vi "Get Connector Pane Info.vi"(8 "error in (no error)":errorcluster, 11 "vi reference":refnum<vi>) -> (0 "error out":errorcluster, 3 "Terminals":T1[](array[typedef]))   [LabVIEW 2020, in "MCP Server.lvlib"]
doc: "Utilizes the Application method \"Get ConPane Datatype\" to read the terminal properties of a subVI without loading it or requiring VI scripting."
uses:
  MCP Server.lvlib
  <vilib>/Utility/Data Type/NI_Data Type.lvlib
  Terminal.ctl
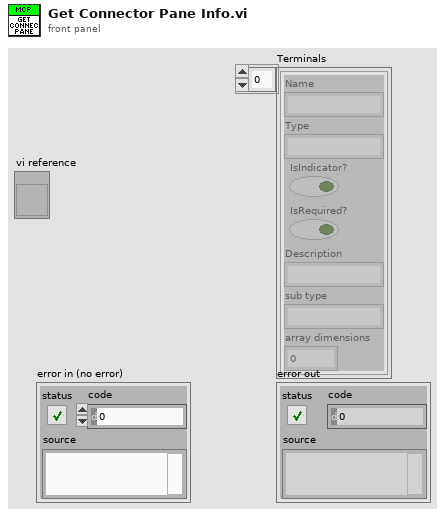
[diagram p1: front panel]
types:
  T1 = typedef "MCP Server.lvlib/Terminal.ctl" = cluster{"Name":string, "Type":string, "IsIndicator?":bool, "IsRequired?":bool, "Description":string, "sub type":string, "array dimensions":i32}
  T2 = typedef "NI_Data Type.lvlib/VI Info.ctl" = cluster{"Connector Pane Pattern":i16, "Connector Pane Rotation":i16, "Flags":u32[], "Modification Date":timestamp, "Asynchronous":bool, "Non-Function":bool, "Subroutine":bool, "SubSystem":bool}
  T3 = typedef "NI_Data Type.lvlib/Data Type.ctl" = enum8{"Invalid Type", "Void", "I8", "I16", "I32", "I64", "U8", "U16", "U32", "U64", "Single Float", "Double Float", "Extended Float", "Single Complex", "Double Complex", "Extended Complex", "Enum U8", "Enum U16", "Enum U32", "Enum U64", "Single Float With Unit", "Double Float With Unit", "Extended Float With Unit", "Single Complex with Unit", "Double Complex with Unit", "Extended Complex with Unit", "Boolean", "String", "Path", "Picture", "Tag", "Array", "Cluster", "Variant", "LV Variant", "Waveform", "Timestamp", "Digital Waveform", "Digital Data", "ExpressData", "Refnum", "External Data", "VI", "Poly VI", "LabVIEW Class Instance", "Fixed Point", "Set Collection", "Map Collection"}
  T4 = typedef "NI_Data Type.lvlib/Memory Info.ctl" = cluster{"Type":T5, "Size":u32}
  T5 = typedef "NI_Data Type.lvlib/Memory Type.ctl" = enum16{"Variable", "Fixed", "Bounded"}
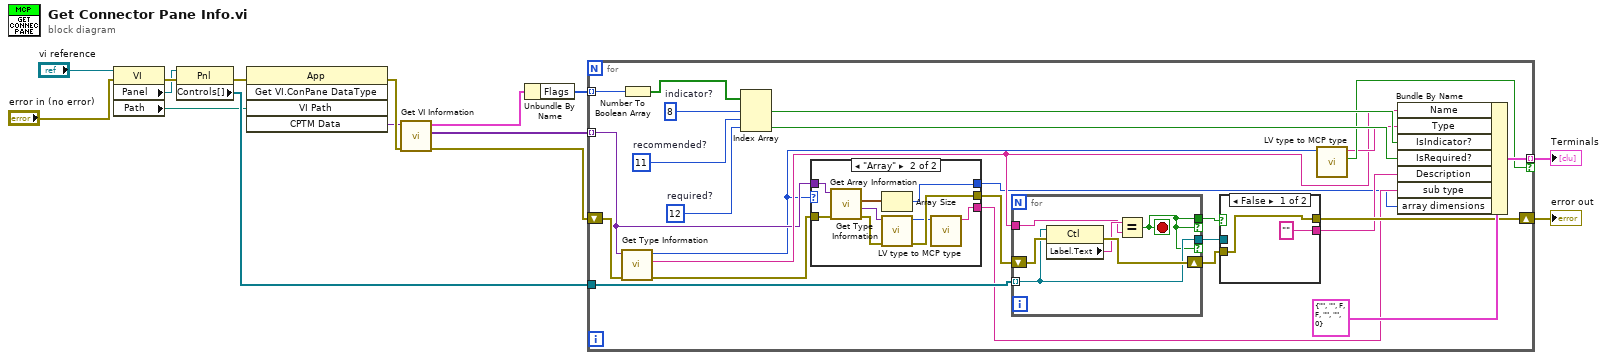
[diagram p0: block diagram]
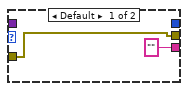
[diagram p2: hidden frame]
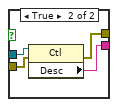
[diagram p3: hidden frame]
diagram:
  n1 = property class="VI"(reference="vi reference", error in="error in (no error)") -> (error out=w6:errorcluster, "Panel"=w4:refnum<vi>, "Path"=w1:path)  [unwired: 1 out]
  n2 = property class="Pnl"(reference=w4, error in=w6) -> (error out=w5:errorcluster, "Controls[]"=w3:refnum<vi>[])  [unwired: 1 out]
  n3 = invoke class="App" method="Get VI.ConPane DataType"(error in=w5, "VI Path"=w1) -> (error out=w12:errorcluster, "CPTM Data"=w8:variant)  [unwired: 3 in, 3 out]
  n4 = call <vilib>:"Get VI Information.vi"("error in (no error)"=w12, "variant"=w8) -> ("error out"=w11:errorcluster, "VI terminal types"=w7:variant[], "VI info"=w9:T2)  [unwired: 6 in, 1 out]
  n5 = Unbundle By Name(w9) -> ("Flags"=w10:u32[])
  n6 = for {
    tunnel: w7 -> [w19] mode=indexing
    tunnel: w10 -> [w40] mode=indexing
    shift-right: [w25] -> w14
    shift-left: w11 -> [w34]
    tunnel: [w30] -> w15 mode=indexing if=w29
    tunnel: w3 -> [w26]
    w36 = 12  # required?
    w37 = 11  # recommended?
    w38 = 8  # indicator?
    n7 = call <vilib>:"Get Type Information.vi"("error in (no error)"=w34, "variant"=w19) -> ("error out"=w35:errorcluster, "name"=w20:string, "type"=w16:T3)  [unwired: 5 in, 2 out]
    n8 = Number To Boolean Array(number=w40) -> (Boolean array=w39:bool[])
    n9 = Index Array(array=w39, index #1=w38, index #2=w37, index #3=w36) -> (element #1=w32:bool, element #3=w31:bool)  [unwired: 1 out]
    n10 = case shown="\"Array\"" w16 {
      tunnel: w35 -> [w42 w51]
      tunnel: [w42 w48] -> w21
      tunnel: w19 -> [_ w49]
      tunnel: ["" ("JSON to Insert") w45] -> w18
      tunnel: [_ w43] -> w17
      frame Default {
      }
      frame "Array" {
        n11 = call <vilib>:"Get Array Information.vi"("error in (no error)"=w51, "variant"=w49) -> ("error out"=w50:errorcluster, "array element data type"=w47:variant, "array lengths"=w44:T4[])  [unwired: 6 in, 1 out]
        n12 = Array Size(array=w44) -> (size(s)=w43:i32)
        n13 = call <vilib>:"Get Type Information.vi"("error in (no error)"=w50, "variant"=w47) -> ("error out"=w48:errorcluster, "type"=w46:T3)  [unwired: 5 in, 3 out]
        n14 = call "LV type to MCP type.vi"("type"=w46) -> ("JSON to Insert"=w45:string)  [unwired: 9 in, 1 out]
      }
    }
    n15 = for {
      tunnel: w26 -> [w59] mode=indexing
      tunnel: w20 -> [w60]
      shift-right: [w62] -> w27
      shift-left: w21 -> [w63]
      tunnel: [w59] -> w24 if=w58
      tunnel: [w58] -> w22 if=w58
      stop <- w58 stop-if-true
      n16 = property class="Ctl"(reference=w59, error in=w63) -> (error out=w62:errorcluster, "Label.Text"=w61:string)  [unwired: 1 out]
      n17 = Equal?(x=w61, y=w60) -> (x = y?=w58:bool)
    }
    n18 = case shown="False" w22 {
      tunnel: w27 -> [w53 w57]
      tunnel: [w53 w56] -> w25
      tunnel: w24 -> [_ w55]
      tunnel: ["" ("Desc") w54] -> w23
      frame False {
      }
      frame True {
        n19 = property class="Ctl"(reference=w55, error in=w57) -> (error out=w56:errorcluster, "Desc"=w54:string)  [unwired: 1 out]
      }
    }
    n20 = call "LV type to MCP type.vi"("type"=w16) -> ("Valid?"=w29:bool, "JSON to Insert"=w28:string)  [unwired: 9 in]
    n21 = Bundle By Name(cluster=T1 {"Name"="", "Type"="", "IsIndicator?"=FALSE, "IsRequired?"=FALSE, "Description"="", "sub type"="", "array dimensions"=0} ("Terminal"), "Name"=w20, "Type"=w28, "IsIndicator?"=w32, "IsRequired?"=w31, "Description"=w23, "sub type"=w18, "array dimensions"=w17) -> (w30:T1)
  }
  "Terminals" <- w15
  "error out" <- w14
